vi "write_params.vi"(8 "error in (no error)":errorcluster, 10 "params":T1={"base_estimator"="", "n_estimators"=50.0, "learning_rate"=1.0, "algorithm"="SAMME.R", "random_state"=0.0}, 11 "AdaBoostClassifier in":refnum<class "AdaBoostClassifier.lvclass">) -> (0 "error out":errorcluster, 3 "AdaBoostClassifier out":refnum<class "AdaBoostClassifier.lvclass">)   [LabVIEW 2020, in "AdaBoostClassifier.lvclass"]
uses:
  AdaBoostClassifier.lvclass
  Controls/adaboostclassifier_params.ctl
  AdaBoostClassifier.lvclass/AdaBoostClassifier.ctl
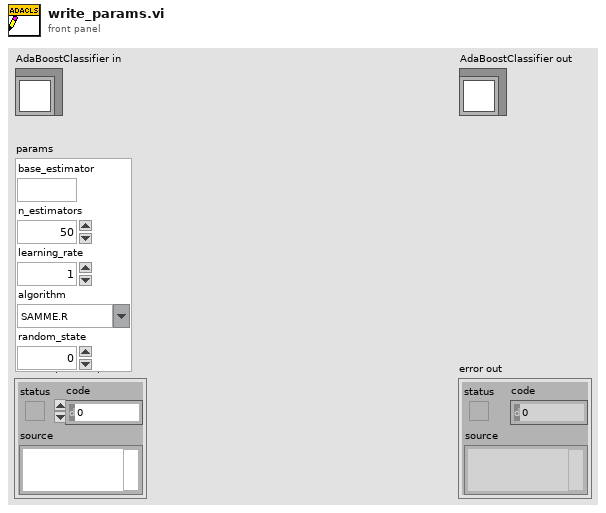
[diagram p1: front panel]
types:
  T1 = typedef "adaboostclassifier_params.ctl" = cluster{"base_estimator":string, "n_estimators":dbl, "learning_rate":dbl, "algorithm":string, "random_state":dbl}
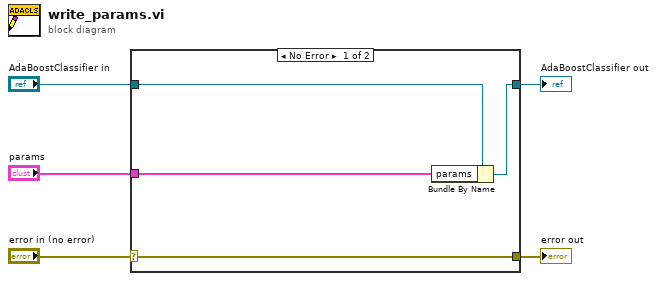
[diagram p0: block diagram]
diagram:
  n1 = case shown="No Error" "error in (no error)" {
    selector: "error in (no error)" -> [w9 w10]
    tunnel: [w9 w10] -> w4
    tunnel: [w7 w11] -> w2
    tunnel: "AdaBoostClassifier in" -> [w8 w11]
    tunnel: "params" -> [w6 _]
    frame No Error {
      n2 = Bundle By Name(cluster=w8, "params"=w6) -> (w7:refnum<class "AdaBoostClassifier.lvclass">)
    }
    frame Error {
    }
  }
  "error out" <- w4
  "AdaBoostClassifier out" <- w2
